vi "Open Connection to All - Type Code Single - Ver 2.vi"(8 "Error In":errorcluster, 10 "Type Code in":i32, 11 "URL":string) -> (0 "Error Out":errorcluster, 1 "Error Status":bool, 2 "Type Code out":i32, 3 "Variable Refnum":variant)   [LabVIEW 2014]
doc: "<B>Copyright</B>: (c) MHWirth 2015. All rights reserved.\n\nThis VI opens connection to all shared variables that are specified using URL and Type arrays. It converts the refnum to variant and send it out.\n\nIf the type is unknown (Error 7001) or read variable function is errorenous, the loop stops and Error Status is True. \n\n<B>Defined Types</B>:\nCode 1. Boolean\nCode 2 to 5. Int8/16/32/64\nCode 6 to 9. UInt8/16/32/64\nCode 10. Double\nCode 11. Single-precision\nCode 12. String\nCode 13 to 24. 1D array of xxx\nCode 25 to 36. 2D array of xxxs\n\n<B>Error 7001</B>: Unknown Data Type - Type Code Array (Int32) contains -1 indicating an unknown data type."
uses:
  Variable Refnum Cluster.ctl
panel:
  out "Cluster of Variavle Refnums":T1
  out "Status":string
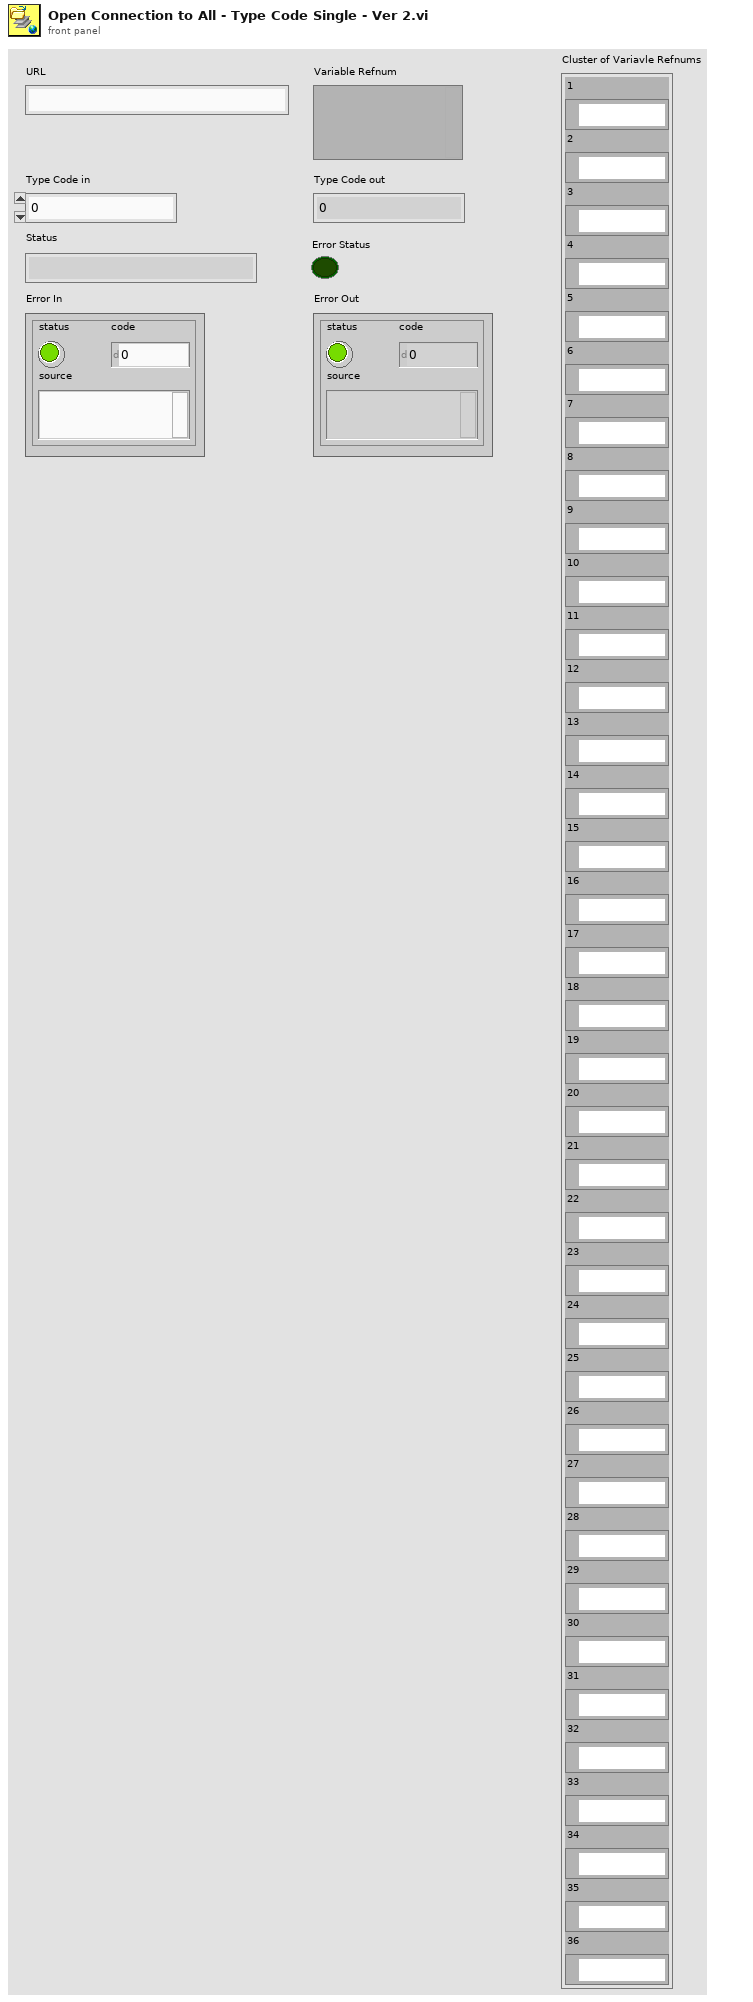
[diagram p1: front panel]
types:
  T1 = typedef "Variable Refnum Cluster.ctl" = cluster{"1":refnum<k21>, "2":refnum<k21>, "3":refnum<k21>, "4":refnum<k21>, "5":refnum<k21>, "6":refnum<k21>, "7":refnum<k21>, "8":refnum<k21>, "9":refnum<k21>, "10":refnum<k21>, "11":refnum<k21>, "12":refnum<k21>, "13":refnum<k21>, "14":refnum<k21>, "15":refnum<k21>, "16":refnum<k21>, "17":refnum<k21>, "18":refnum<k21>, "19":refnum<k21>, "20":refnum<k21>, "21":refnum<k21>, "22":refnum<k21>, "23":refnum<k21>, "24":refnum<k21>, "25":refnum<k21>, "26":refnum<k21>, "27":refnum<k21>, "28":refnum<k21>, "29":refnum<k21>, "30":refnum<k21>, "31":refnum<k21>, "32":refnum<k21>, "33":refnum<k21>, "34":refnum<k21>, "35":refnum<k21>, "36":refnum<k21>}
  T2 = cluster{"shared variable refnum out":refnum<k21>, "shared variable refnum out":refnum<k21>, "shared variable refnum out":refnum<k21>, "shared variable refnum out":refnum<k21>, "shared variable refnum out":refnum<k21>, "shared variable refnum out":refnum<k21>, "shared variable refnum out":refnum<k21>, "shared variable refnum out":refnum<k21>, "shared variable refnum out":refnum<k21>, "shared variable refnum out":refnum<k21>, "shared variable refnum out":refnum<k21>, "shared variable refnum out":refnum<k21>, "shared variable refnum out":refnum<k21>, "shared variable refnum out":refnum<k21>, "shared variable refnum out":refnum<k21>, "shared variable refnum out":refnum<k21>, "shared variable refnum out":refnum<k21>, "shared variable refnum out":refnum<k21>, "shared variable refnum out":refnum<k21>, "shared variable refnum out":refnum<k21>, "shared variable refnum out":refnum<k21>, "shared variable refnum out":refnum<k21>, "shared variable refnum out":refnum<k21>, "shared variable refnum out":refnum<k21>, "shared variable refnum out":refnum<k21>, "shared variable refnum out":refnum<k21>, "shared variable refnum out":refnum<k21>, "shared variable refnum out":refnum<k21>, "shared variable refnum out":refnum<k21>, "shared variable refnum out":refnum<k21>, "shared variable refnum out":refnum<k21>, "shared variable refnum out":refnum<k21>, "shared variable refnum out":refnum<k21>, "shared variable refnum out":refnum<k21>, "shared variable refnum out":refnum<k21>, "shared variable refnum out":refnum<k21>}
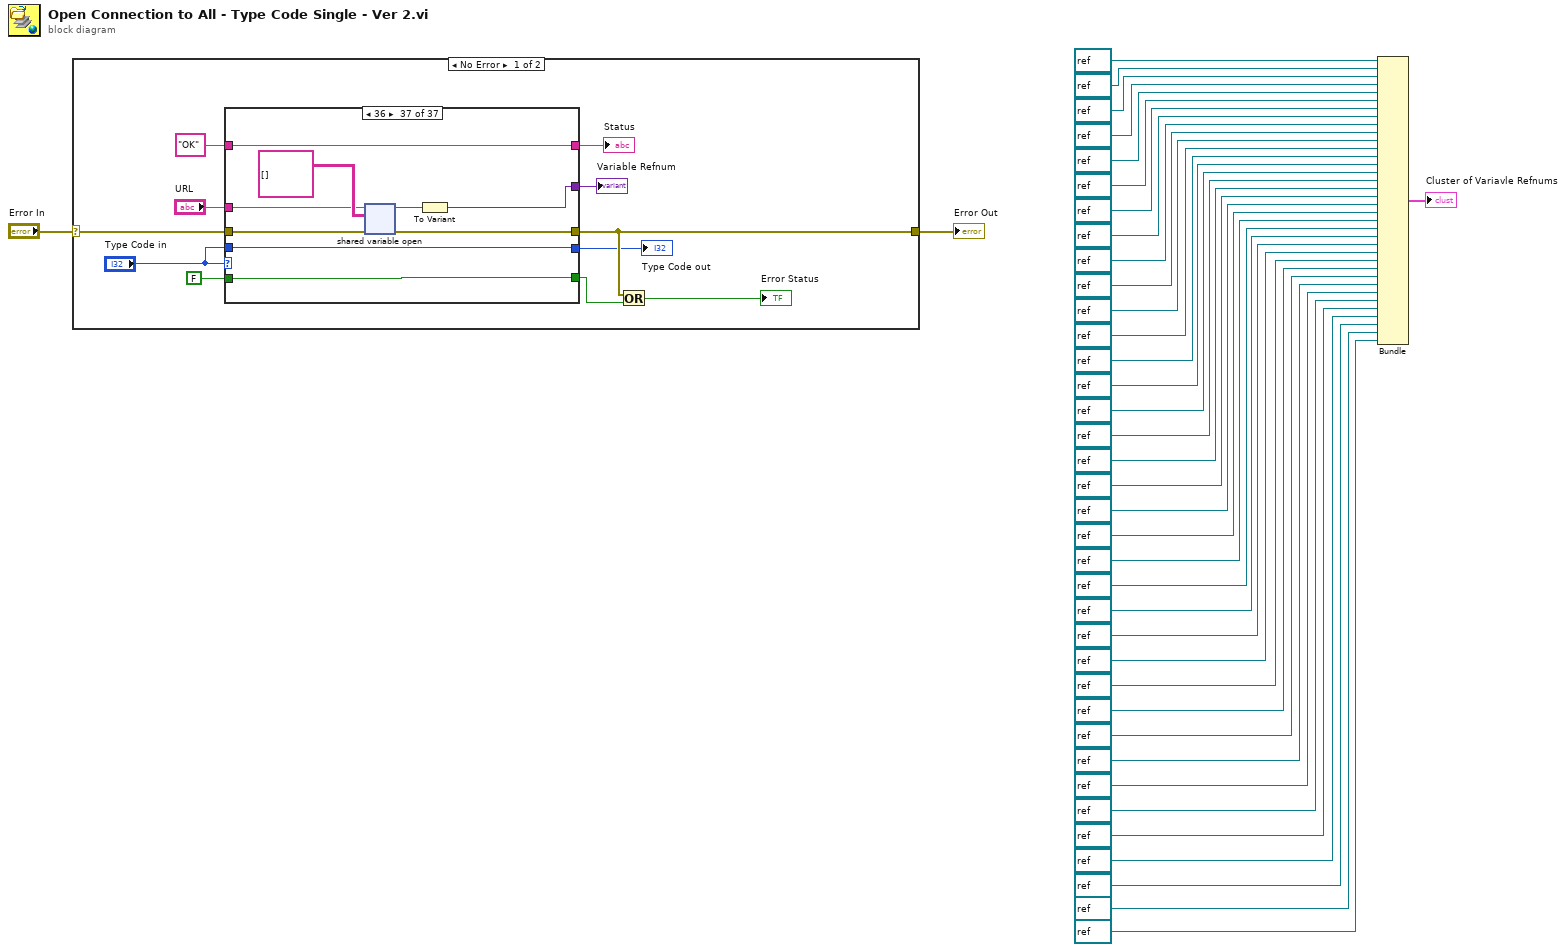
[diagram p0: block diagram]
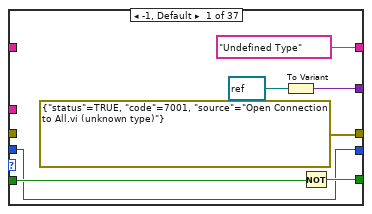
[diagram p2: hidden frame]
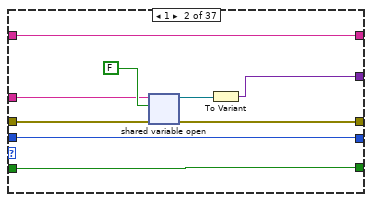
[diagram p3: hidden frame]
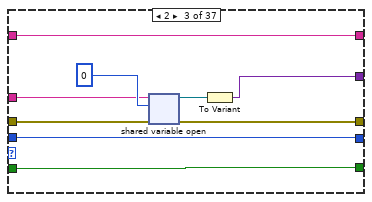
[diagram p4: hidden frame]
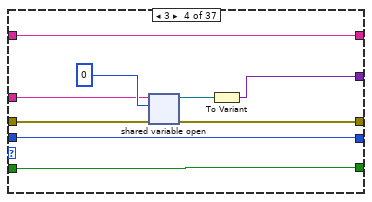
[diagram p5: hidden frame]
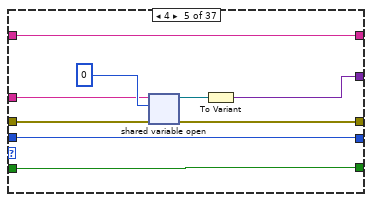
[diagram p6: hidden frame]
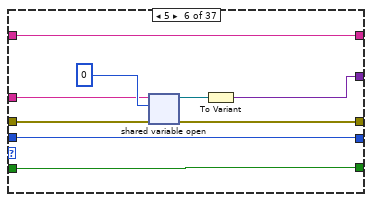
[diagram p7: hidden frame]
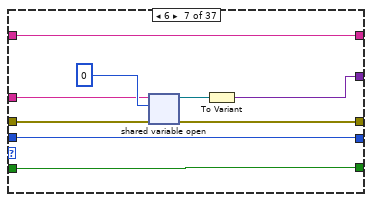
[diagram p8: hidden frame]
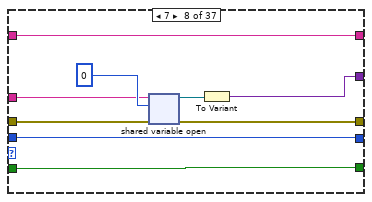
[diagram p9: hidden frame]
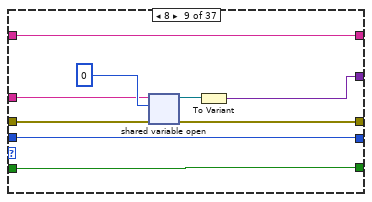
[diagram p10: hidden frame]
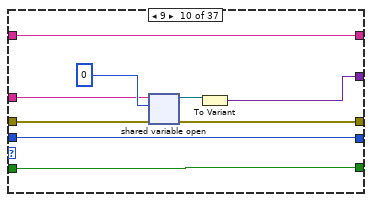
[diagram p11: hidden frame]
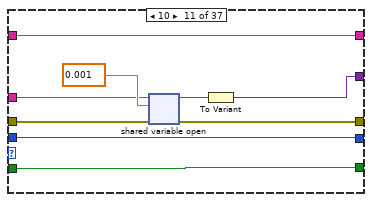
[diagram p12: hidden frame]
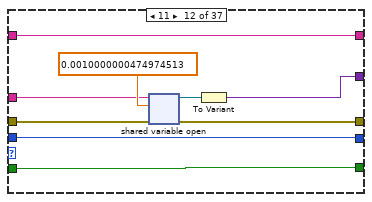
[diagram p13: hidden frame]
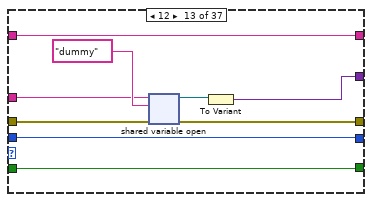
[diagram p14: hidden frame]
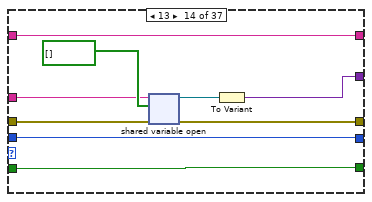
[diagram p15: hidden frame]
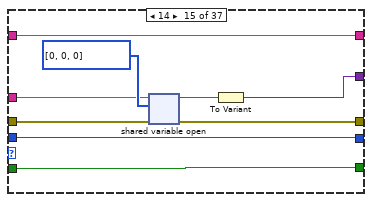
[diagram p16: hidden frame]
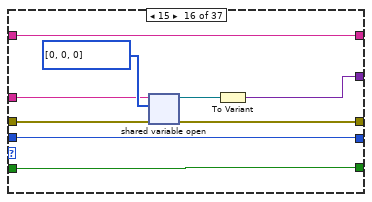
[diagram p17: hidden frame]
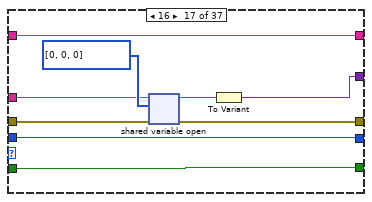
[diagram p18: hidden frame]
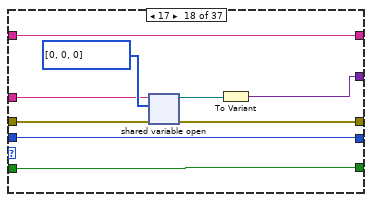
[diagram p19: hidden frame]
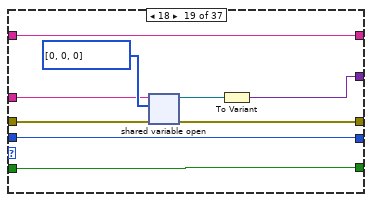
[diagram p20: hidden frame]
diagram:
  n1 = case shown="No Error" "Error In" {
    selector: "Error In" -> [w50 w382]
    tunnel: [w49 w382] -> w38
    frame No Error {
      n2 = case shown="36" "Type Code in" {
        tunnel: w50 -> [_ w65 w74 w83 w92 w101 w110 w119 w128 w137 w146 w155 w165 w173 w182 w191 w200 w209 w218 w227 w236 w245 w254 w263 w272 w281 w290 w299 w308 w317 w326 w335 w344 w353 w362 w371 w380]
        tunnel: [errorcluster {"status"=TRUE, "code"=7001, "source"="Open Connection to All.vi (unknown type)"} ("error constant") w62 w71 w80 w89 w98 w107 w116 w125 w134 w143 w152 w161 w170 w179 w188 w197 w206 w215 w224 w233 w242 w250 w260 w269 w278 w287 w296 w305 w314 w323 w332 w341 w350 w359 w368 w377] -> w49
        tunnel: ["Undefined Type" w64 w73 w82 w91 w100 w109 w118 w127 w136 w145 w154 w164 w172 w181 w190 w199 w208 w217 w226 w235 w244 w253 w262 w271 w280 w289 w298 w307 w316 w325 w334 w343 w352 w361 w370 w379] -> w48
        tunnel: "OK" -> [_ w64 w73 w82 w91 w100 w109 w118 w127 w136 w145 w154 w164 w172 w181 w190 w199 w208 w217 w226 w235 w244 w253 w262 w271 w280 w289 w298 w307 w316 w325 w334 w343 w352 w361 w370 w379]
        tunnel: FALSE -> [w56 w63 w72 w81 w90 w99 w108 w117 w126 w135 w144 w153 w163 w171 w180 w189 w198 w207 w216 w225 w234 w243 w252 w261 w270 w279 w288 w297 w306 w315 w324 w333 w342 w351 w360 w369 w378]
        tunnel: [w55 w63 w72 w81 w90 w99 w108 w117 w126 w135 w144 w153 w163 w171 w180 w189 w198 w207 w216 w225 w234 w243 w252 w261 w270 w279 w288 w297 w306 w315 w324 w333 w342 w351 w360 w369 w378] -> w45
        tunnel: "URL" -> [_ w61 w70 w79 w88 w97 w106 w115 w124 w133 w142 w151 w160 w169 w178 w187 w196 w205 w214 w223 w232 w241 w251 w259 w268 w277 w286 w295 w304 w313 w322 w331 w340 w349 w358 w367 w376]
        tunnel: [w52 w59 w68 w77 w86 w95 w104 w113 w122 w131 w140 w149 w158 w167 w176 w185 w194 w203 w212 w221 w230 w239 w248 w257 w266 w274 w283 w292 w301 w310 w319 w328 w337 w346 w355 w364 w373] -> w42
        tunnel: "Type Code in" -> [w51 w58 w67 w76 w85 w94 w103 w112 w121 w130 w139 w148 w157 w166 w175 w184 w193 w202 w211 w220 w229 w238 w247 w256 w265 w276 w285 w294 w303 w312 w321 w330 w339 w348 w357 w366 w375]
        tunnel: [w51 w58 w67 w76 w85 w94 w103 w112 w121 w130 w139 w148 w157 w166 w175 w184 w193 w202 w211 w220 w229 w238 w247 w256 w265 w276 w285 w294 w303 w312 w321 w330 w339 w348 w357 w366 w375] -> w40
        frame -1, Default {
          n3 = To Variant(anything=refnum<k21> refnum) -> (Variant=w52:variant)
          n4 = Not(x=w56) -> (.not. x?=w55:bool)
        }
        frame 1 {
          n5 = shared-variable-open(w61, w65, FALSE) -> (w60:refnum<k21>, w62:errorcluster)  [unwired: 1 in]
          n6 = To Variant(anything=w60) -> (Variant=w59:variant)
        }
        frame 2 {
          n7 = shared-variable-open(w70, w74, i8 0) -> (w69:refnum<k21>, w71:errorcluster)  [unwired: 1 in]
          n8 = To Variant(anything=w69) -> (Variant=w68:variant)
        }
        frame 3 {
          n9 = shared-variable-open(w79, w83, i16 0) -> (w78:refnum<k21>, w80:errorcluster)  [unwired: 1 in]
          n10 = To Variant(anything=w78) -> (Variant=w77:variant)
        }
        frame 4 {
          n11 = shared-variable-open(w88, w92, 0) -> (w87:refnum<k21>, w89:errorcluster)  [unwired: 1 in]
          n12 = To Variant(anything=w87) -> (Variant=w86:variant)
        }
        frame 5 {
          n13 = shared-variable-open(w97, w101, i64 0) -> (w96:refnum<k21>, w98:errorcluster)  [unwired: 1 in]
          n14 = To Variant(anything=w96) -> (Variant=w95:variant)
        }
        frame 6 {
          n15 = shared-variable-open(w106, w110, u8 0) -> (w105:refnum<k21>, w107:errorcluster)  [unwired: 1 in]
          n16 = To Variant(anything=w105) -> (Variant=w104:variant)
        }
        frame 7 {
          n17 = shared-variable-open(w115, w119, u16 0) -> (w114:refnum<k21>, w116:errorcluster)  [unwired: 1 in]
          n18 = To Variant(anything=w114) -> (Variant=w113:variant)
        }
        frame 8 {
          n19 = shared-variable-open(w124, w128, u32 0) -> (w123:refnum<k21>, w125:errorcluster)  [unwired: 1 in]
          n20 = To Variant(anything=w123) -> (Variant=w122:variant)
        }
        frame 9 {
          n21 = shared-variable-open(w133, w137, u64 0) -> (w132:refnum<k21>, w134:errorcluster)  [unwired: 1 in]
          n22 = To Variant(anything=w132) -> (Variant=w131:variant)
        }
        frame 10 {
          n23 = shared-variable-open(w142, w146, 0.001) -> (w141:refnum<k21>, w143:errorcluster)  [unwired: 1 in]
          n24 = To Variant(anything=w141) -> (Variant=w140:variant)
        }
        frame 11 {
          n25 = shared-variable-open(w151, w155, sgl 0.001) -> (w150:refnum<k21>, w152:errorcluster)  [unwired: 1 in]
          n26 = To Variant(anything=w150) -> (Variant=w149:variant)
        }
        frame 12 {
          n27 = shared-variable-open(w160, w165, "dummy") -> (w159:refnum<k21>, w161:errorcluster)  [unwired: 1 in]
          n28 = To Variant(anything=w159) -> (Variant=w158:variant)
        }
        frame 13 {
          n29 = shared-variable-open(w169, w173, bool[] []) -> (w168:refnum<k21>, w170:errorcluster)  [unwired: 1 in]
          n30 = To Variant(anything=w168) -> (Variant=w167:variant)
        }
        frame 14 {
          n31 = shared-variable-open(w178, w182, i8[] [0, 0, 0]) -> (w177:refnum<k21>, w179:errorcluster)  [unwired: 1 in]
          n32 = To Variant(anything=w177) -> (Variant=w176:variant)
        }
        frame 15 {
          n33 = shared-variable-open(w187, w191, i16[] [0, 0, 0]) -> (w186:refnum<k21>, w188:errorcluster)  [unwired: 1 in]
          n34 = To Variant(anything=w186) -> (Variant=w185:variant)
        }
        frame 16 {
          n35 = shared-variable-open(w196, w200, i32[] [0, 0, 0]) -> (w195:refnum<k21>, w197:errorcluster)  [unwired: 1 in]
          n36 = To Variant(anything=w195) -> (Variant=w194:variant)
        }
        frame 17 {
          n37 = shared-variable-open(w205, w209, i64[] [0, 0, 0]) -> (w204:refnum<k21>, w206:errorcluster)  [unwired: 1 in]
          n38 = To Variant(anything=w204) -> (Variant=w203:variant)
        }
        frame 18 {
          n39 = shared-variable-open(w214, w218, u8[] [0, 0, 0]) -> (w213:refnum<k21>, w215:errorcluster)  [unwired: 1 in]
          n40 = To Variant(anything=w213) -> (Variant=w212:variant)
        }
        frame 19 {
          n41 = shared-variable-open(w223, w227, u16[] [0, 0, 0]) -> (w222:refnum<k21>, w224:errorcluster)  [unwired: 1 in]
          n42 = To Variant(anything=w222) -> (Variant=w221:variant)
        }
        frame 20 {
          n43 = shared-variable-open(w232, w236, u32[] [0, 0, 0]) -> (w231:refnum<k21>, w233:errorcluster)  [unwired: 1 in]
          n44 = To Variant(anything=w231) -> (Variant=w230:variant)
        }
        frame 21 {
          n45 = shared-variable-open(w241, w245, u64[] [0, 0, 0]) -> (w240:refnum<k21>, w242:errorcluster)  [unwired: 1 in]
          n46 = To Variant(anything=w240) -> (Variant=w239:variant)
        }
        frame 22 {
          n47 = shared-variable-open(w251, w254, dbl[] [0.0, 0.0, 0.0]) -> (w249:refnum<k21>, w250:errorcluster)  [unwired: 1 in]
          n48 = To Variant(anything=w249) -> (Variant=w248:variant)
        }
        frame 23 {
          n49 = shared-variable-open(w259, w263, sgl[] [0.0, 0.0, 0.0]) -> (w258:refnum<k21>, w260:errorcluster)  [unwired: 1 in]
          n50 = To Variant(anything=w258) -> (Variant=w257:variant)
        }
        frame 24 {
          n51 = shared-variable-open(w268, w272, string[] []) -> (w267:refnum<k21>, w269:errorcluster)  [unwired: 1 in]
          n52 = To Variant(anything=w267) -> (Variant=w266:variant)
        }
        frame 25 {
          n53 = shared-variable-open(w277, w281, bool[][] []) -> (w275:refnum<k21>, w278:errorcluster)  [unwired: 1 in]
          n54 = To Variant(anything=w275) -> (Variant=w274:variant)
        }
        frame 26 {
          n55 = shared-variable-open(w286, w290, i8[][] [[0, 0, 0]]) -> (w284:refnum<k21>, w287:errorcluster)  [unwired: 1 in]
          n56 = To Variant(anything=w284) -> (Variant=w283:variant)
        }
        frame 27 {
          n57 = shared-variable-open(w295, w299, i16[][] [[0, 0, 0]]) -> (w293:refnum<k21>, w296:errorcluster)  [unwired: 1 in]
          n58 = To Variant(anything=w293) -> (Variant=w292:variant)
        }
        frame 28 {
          n59 = shared-variable-open(w304, w308, i32[][] [[0, 0, 0]]) -> (w302:refnum<k21>, w305:errorcluster)  [unwired: 1 in]
          n60 = To Variant(anything=w302) -> (Variant=w301:variant)
        }
        frame 29 {
          n61 = shared-variable-open(w313, w317, i64[][] [[0, 0, 0]]) -> (w311:refnum<k21>, w314:errorcluster)  [unwired: 1 in]
          n62 = To Variant(anything=w311) -> (Variant=w310:variant)
        }
        frame 30 {
          n63 = shared-variable-open(w322, w326, u8[][] [[0, 0, 0]]) -> (w320:refnum<k21>, w323:errorcluster)  [unwired: 1 in]
          n64 = To Variant(anything=w320) -> (Variant=w319:variant)
        }
        frame 31 {
          n65 = shared-variable-open(w331, w335, u16[][] [[0, 0, 0]]) -> (w329:refnum<k21>, w332:errorcluster)  [unwired: 1 in]
          n66 = To Variant(anything=w329) -> (Variant=w328:variant)
        }
        frame 32 {
          n67 = shared-variable-open(w340, w344, u32[][] [[0, 0, 0]]) -> (w338:refnum<k21>, w341:errorcluster)  [unwired: 1 in]
          n68 = To Variant(anything=w338) -> (Variant=w337:variant)
        }
        frame 33 {
          n69 = shared-variable-open(w349, w353, u64[][] [[0, 0, 0]]) -> (w347:refnum<k21>, w350:errorcluster)  [unwired: 1 in]
          n70 = To Variant(anything=w347) -> (Variant=w346:variant)
        }
        frame 34 {
          n71 = shared-variable-open(w358, w362, dbl[][] [[0.0, 0.0, 0.0]]) -> (w356:refnum<k21>, w359:errorcluster)  [unwired: 1 in]
          n72 = To Variant(anything=w356) -> (Variant=w355:variant)
        }
        frame 35 {
          n73 = shared-variable-open(w367, w371, sgl[][] [[0.0, 0.0, 0.0]]) -> (w365:refnum<k21>, w368:errorcluster)  [unwired: 1 in]
          n74 = To Variant(anything=w365) -> (Variant=w364:variant)
        }
        frame 36 {
          n75 = shared-variable-open(w376, w380, string[][] []) -> (w374:refnum<k21>, w377:errorcluster)  [unwired: 1 in]
          n76 = To Variant(anything=w374) -> (Variant=w373:variant)
        }
      }
      "Status" <- w48
      "Type Code out" <- w40
      "Variable Refnum" <- w42
      n77 = Or(x=w49, y=w45) -> (x .or. y?=→"Error Status":bool)
    }
    frame Error {
    }
  }
  "Error Out" <- w38
  n78 = Bundle("shared variable refnum out"=refnum<k21> refnum, "shared variable refnum out"=refnum<k21> refnum, "shared variable refnum out"=refnum<k21> refnum, "shared variable refnum out"=refnum<k21> refnum, "shared variable refnum out"=refnum<k21> refnum, "shared variable refnum out"=refnum<k21> refnum, "shared variable refnum out"=refnum<k21> refnum, "shared variable refnum out"=refnum<k21> refnum, "shared variable refnum out"=refnum<k21> refnum, "shared variable refnum out"=refnum<k21> refnum, "shared variable refnum out"=refnum<k21> refnum, "shared variable refnum out"=refnum<k21> refnum, "shared variable refnum out"=refnum<k21> refnum, "shared variable refnum out"=refnum<k21> refnum, "shared variable refnum out"=refnum<k21> refnum, "shared variable refnum out"=refnum<k21> refnum, "shared variable refnum out"=refnum<k21> refnum, "shared variable refnum out"=refnum<k21> refnum, "shared variable refnum out"=refnum<k21> refnum, "shared variable refnum out"=refnum<k21> refnum, "shared variable refnum out"=refnum<k21> refnum, "shared variable refnum out"=refnum<k21> refnum, "shared variable refnum out"=refnum<k21> refnum, "shared variable refnum out"=refnum<k21> refnum, "shared variable refnum out"=refnum<k21> refnum, "shared variable refnum out"=refnum<k21> refnum, "shared variable refnum out"=refnum<k21> refnum, "shared variable refnum out"=refnum<k21> refnum, "shared variable refnum out"=refnum<k21> refnum, "shared variable refnum out"=refnum<k21> refnum, "shared variable refnum out"=refnum<k21> refnum, "shared variable refnum out"=refnum<k21> refnum, "shared variable refnum out"=refnum<k21> refnum, "shared variable refnum out"=refnum<k21> refnum, "shared variable refnum out"=refnum<k21> refnum, "shared variable refnum out"=refnum<k21> refnum) -> (→"Cluster of Variavle Refnums":T2)  [unwired: 1 in]
